vi "Send2Cerebus32.vi"(4 "ErrorIn":errorcluster, 5 "String":string, 7 "Mode":T1(ring)) -> (0 "ErrorOut":errorcluster)   [LabVIEW 2013]
uses:
  <vilib>/DAQmx/write.llb/DAQmx Write (Digital 1D Bool 1Chan 1Samp).vi
  <vilib>/DAQmx/miscellaneous.llb/DAQmx Fill In Error Info.vi
  <resource>/objmgr/daqmx.rc
panel:
  out "TaskID":refnum<k21>="cerebus_markers"
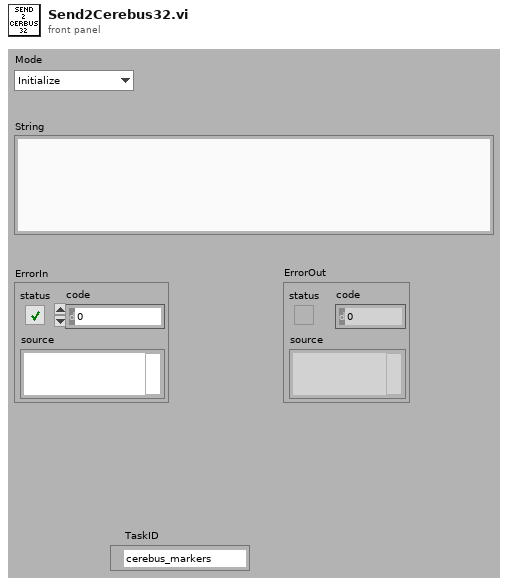
[diagram p1: front panel]
types:
  T1 = enum16{"Initialize", "String", "Start", "Stop", "Close"}
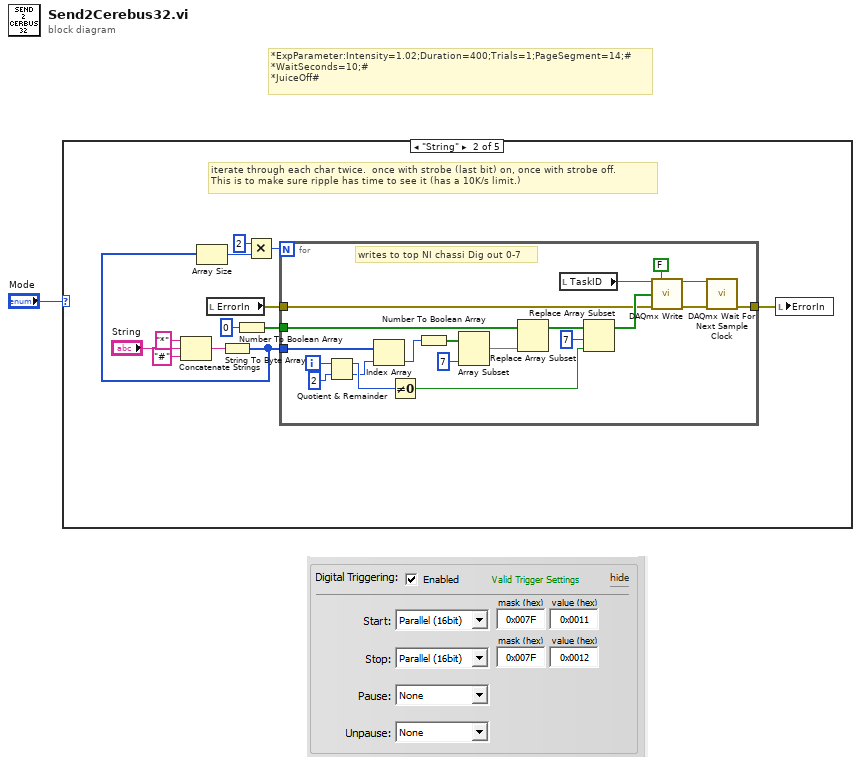
[diagram p0: block diagram]
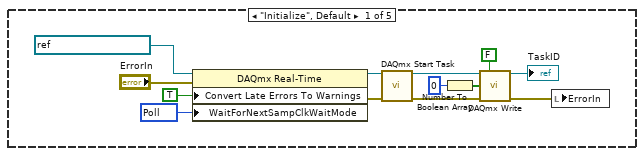
[diagram p2: hidden frame]
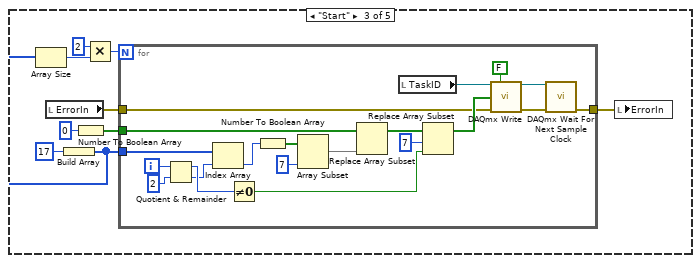
[diagram p3: hidden frame]
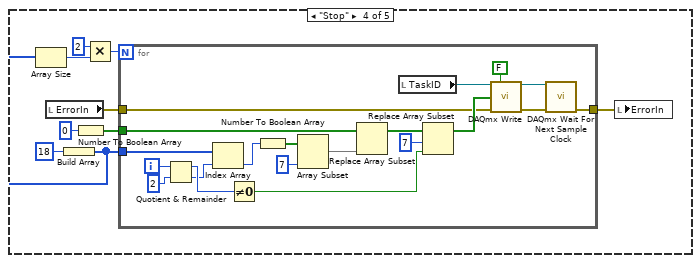
[diagram p4: hidden frame]
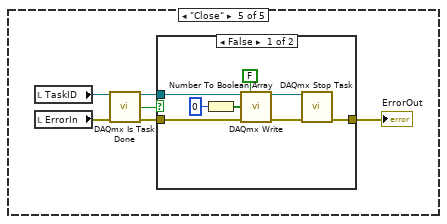
[diagram p5: hidden frame]
diagram:
  # "*ExpParameter:Intensity=1.02;Duration=400;Trials=1;PageSegment=14;#\n*WaitSeconds=10;#\n*JuiceOff#"
  n1 = case shown="\"String\"" "Mode" {
    frame "Initialize", Default {
      w3 = 12524 items=["Wait For Interrupt"=12523, "Poll"=12524] ("WaitForNextSampClkWaitMode")
      n2 = property class="DAQmx Real-Time"(reference=refnum<k21> "cerebus_markers" ("task/channels in"), error in="ErrorIn", "Convert Late Errors To Warnings"=TRUE ("ConvLateErrorsToWarnings"), "WaitForNextSampClkWaitMode"=w3) -> (reference out=w8:refnum<k21>, error out=w7:errorcluster)
      n3 = call <vilib>:"DAQmx Start Task.vi"("task/channels in"=w8, "error in"=w7) -> ("task out"=w14:refnum<k21>, "error out"=w11:errorcluster)  [unwired: 12 in]
      n4 = Number To Boolean Array(number=u32 0) -> (Boolean array=w12:bool[])
      n5 = call-poly <vilib>:"DAQmx Write.vi"("task/channels in"=w14, "auto start"=FALSE, "data"=w12, "error in"=w11) -> ("task out"=→"TaskID":refnum<k21>, "error out"=w4:errorcluster)  [unwired: 9 in, 1 out]
      n6 = local write "ErrorIn"(w4) -> ()
    }
    frame "String" {
      # "iterate through each char twice.  once with strobe (last bit) on, once with strobe off.  \nThis is to make sure ripple has time to see it (has a 10K/s limit.)"
      n7 = Concatenate Strings("*", "String", "#" ("string")) -> (w24:string)
      n8 = local read "ErrorIn"() -> (w20:errorcluster)
      n9 = String To Byte Array(string=w24) -> (unsigned byte array=w18:u8[])
      n10 = Array Size(array=w18) -> (size(s)=w17:i32)
      n11 = Number To Boolean Array(number=u32 0) -> (Boolean array=w21:bool[])
      n12 = Multiply(x=2, y=w17) -> (x*y=w15:i32)
      n13 = for {
        N: w15 -> [_]
        tunnel: w18 -> [w29]
        tunnel: w21 -> [w42]
        tunnel: w20 -> [w35]
        tunnel: [w36] -> w19
        i -> [w33]
        # "writes to top NI chassi Dig out 0-7"
        n14 = Quotient & Remainder(x=w33, y=2) -> (x-y*floor(x/y)=w31:i32, floor(x/y)=w27:i32)
        n15 = Index Array(array=w29, index=w27) -> (element=w28:u8)
        n16 = Not Equal To 0?(x=w31) -> (x != 0?=w30:bool)
        n17 = Number To Boolean Array(number=w28) -> (Boolean array=w41:bool[])
        n18 = Array Subset(array=w41, length=7) -> (w40:bool[])  [unwired: 1 in]
        n19 = Replace Array Subset(array=w42, new element=w40) -> (w38:bool[])  [unwired: 1 in]
        n20 = local read "TaskID"() -> (w34:refnum<k21>)
        n21 = Replace Array Subset(array=w38, new element=w30, index=7) -> (w37:bool[])
        n22 = call-poly <vilib>:"DAQmx Write.vi"("task/channels in"=w34, "auto start"=FALSE, "data"=w37, "error in"=w35) -> ("task out"=w44:refnum<k21>, "error out"=w43:errorcluster)  [unwired: 9 in, 1 out]
        n23 = call <vilib>:"DAQmx Wait For Next Sample Clock.vi"("task/channels in"=w44, "error in"=w43) -> ("error out"=w36:errorcluster)  [unwired: 11 in, 2 out]
      }
      n24 = local write "ErrorIn"(w19) -> ()
    }
    frame "Start" {
      n25 = local read "ErrorIn"() -> (w53:errorcluster)
      n26 = Build Array(u8 17) -> (w47:u8[])
      n27 = Array Size(array=w47) -> (size(s)=w51:i32)
      n28 = Number To Boolean Array(number=u32 0) -> (Boolean array=w54:bool[])
      n29 = Multiply(x=2, y=w51) -> (x*y=w49:i32)
      n30 = for {
        N: w49 -> [_]
        tunnel: w47 -> [w58]
        tunnel: w54 -> [w71]
        tunnel: w53 -> [w64]
        tunnel: [w65] -> w52
        i -> [w62]
        n31 = Quotient & Remainder(x=w62, y=2) -> (x-y*floor(x/y)=w60:i32, floor(x/y)=w56:i32)
        n32 = Index Array(array=w58, index=w56) -> (element=w57:u8)
        n33 = Not Equal To 0?(x=w60) -> (x != 0?=w59:bool)
        n34 = Number To Boolean Array(number=w57) -> (Boolean array=w70:bool[])
        n35 = Array Subset(array=w70, length=7) -> (w69:bool[])  [unwired: 1 in]
        n36 = Replace Array Subset(array=w71, new element=w69) -> (w67:bool[])  [unwired: 1 in]
        n37 = local read "TaskID"() -> (w63:refnum<k21>)
        n38 = Replace Array Subset(array=w67, new element=w59, index=7) -> (w66:bool[])
        n39 = call-poly <vilib>:"DAQmx Write.vi"("task/channels in"=w63, "auto start"=FALSE, "data"=w66, "error in"=w64) -> ("task out"=w73:refnum<k21>, "error out"=w72:errorcluster)  [unwired: 9 in, 1 out]
        n40 = call <vilib>:"DAQmx Wait For Next Sample Clock.vi"("task/channels in"=w73, "error in"=w72) -> ("error out"=w65:errorcluster)  [unwired: 11 in, 2 out]
      }
      n41 = local write "ErrorIn"(w52) -> ()
    }
    frame "Stop" {
      n42 = local read "ErrorIn"() -> (w82:errorcluster)
      n43 = Build Array(u8 18) -> (w76:u8[])
      n44 = Array Size(array=w76) -> (size(s)=w80:i32)
      n45 = Number To Boolean Array(number=u32 0) -> (Boolean array=w83:bool[])
      n46 = Multiply(x=2, y=w80) -> (x*y=w78:i32)
      n47 = for {
        N: w78 -> [_]
        tunnel: w76 -> [w87]
        tunnel: w83 -> [w100]
        tunnel: w82 -> [w93]
        tunnel: [w94] -> w81
        i -> [w91]
        n48 = Quotient & Remainder(x=w91, y=2) -> (x-y*floor(x/y)=w89:i32, floor(x/y)=w85:i32)
        n49 = Index Array(array=w87, index=w85) -> (element=w86:u8)
        n50 = Not Equal To 0?(x=w89) -> (x != 0?=w88:bool)
        n51 = Number To Boolean Array(number=w86) -> (Boolean array=w99:bool[])
        n52 = Array Subset(array=w99, length=7) -> (w98:bool[])  [unwired: 1 in]
        n53 = Replace Array Subset(array=w100, new element=w98) -> (w96:bool[])  [unwired: 1 in]
        n54 = local read "TaskID"() -> (w92:refnum<k21>)
        n55 = Replace Array Subset(array=w96, new element=w88, index=7) -> (w95:bool[])
        n56 = call-poly <vilib>:"DAQmx Write.vi"("task/channels in"=w92, "auto start"=FALSE, "data"=w95, "error in"=w93) -> ("task out"=w102:refnum<k21>, "error out"=w101:errorcluster)  [unwired: 9 in, 1 out]
        n57 = call <vilib>:"DAQmx Wait For Next Sample Clock.vi"("task/channels in"=w102, "error in"=w101) -> ("error out"=w94:errorcluster)  [unwired: 11 in, 2 out]
      }
      n58 = local write "ErrorIn"(w81) -> ()
    }
    frame "Close" {
      n59 = local read "TaskID"() -> (w109:refnum<k21>)
      n60 = local read "ErrorIn"() -> (w108:errorcluster)
      n61 = call <vilib>:"DAQmx Is Task Done.vi"("task/channels in"=w109, "error in"=w108) -> ("task out"=w107:refnum<k21>, "task done?"=w105:bool, "error out"=w106:errorcluster)  [unwired: 11 in]
      n62 = case shown="False" w105 {
        tunnel: w107 -> [w115 _]
        tunnel: w106 -> [w112 w119]
        tunnel: [w111 w119] -> w110
        frame False {
          n63 = Number To Boolean Array(number=u32 0) -> (Boolean array=w117:bool[])
          n64 = call-poly <vilib>:"DAQmx Write.vi"("task/channels in"=w115, "auto start"=FALSE, "data"=w117, "error in"=w112) -> ("task out"=w116:refnum<k21>, "error out"=w114:errorcluster)  [unwired: 9 in, 1 out]
          n65 = call <vilib>:"DAQmx Stop Task.vi"("task/channels in"=w116, "error in"=w114) -> ("error out"=w111:errorcluster)  [unwired: 12 in, 1 out]
        }
        frame True {
        }
      }
      "ErrorOut" <- w110
    }
  }
